vi "Change Setpoint.vi"(8 "error in":errorcluster, 10 "Setpoint":dbl, 11 "TE Cooler in":refnum<class "TE Cooler.lvclass">) -> (0 "error out":errorcluster, 3 "TE Cooler out":refnum<class "TE Cooler.lvclass">)   [LabVIEW 2014, in "TE Cooler.lvlib" / "TE Cooler.lvclass"]
uses:
  TE Cooler.lvclass
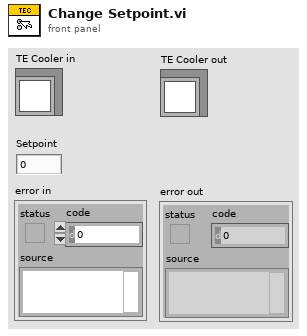
[diagram p1: front panel]
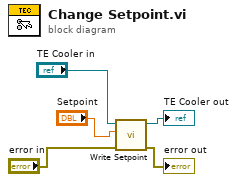
[diagram p0: block diagram]
diagram:
  n1 = call "Write Setpoint.vi"("error in"="error in", "SP"="Setpoint", "TE Cooler in"="TE Cooler in") -> ("error out"=→"error out":errorcluster, "TE Cooler out"=→"TE Cooler out":refnum<class "TE Cooler.lvclass">)  [unwired: 7 in]
